vi "Tests_Window.vi"   [LabVIEW 2024]
uses:
  GLF/Window/Window.lvclass
  GLF/View/View.lvclass
  GLF/Engine/Engine.lvclass
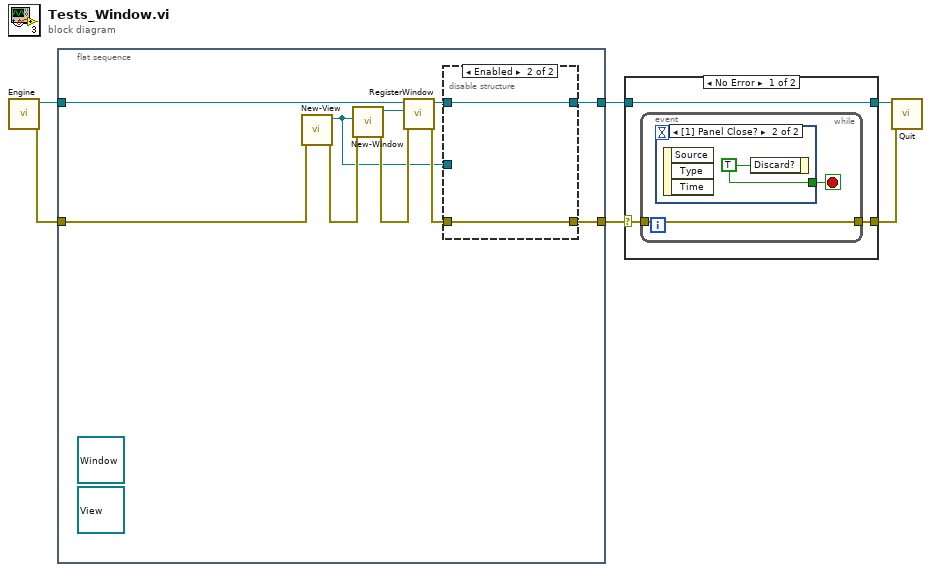
[diagram p0: block diagram]
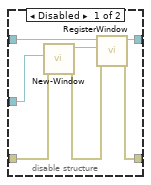
[diagram p2: hidden frame]
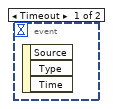
[diagram p3: hidden frame]
diagram:
  n1 = call "Engine.vi"() -> ("error out"=w5:errorcluster, "Engine"=w1:refnum<class "Engine.lvclass">)  [unwired: 10 in]
  n2 = flat-sequence {
    tunnel: w5 -> [w16]
    tunnel: [w8] -> w4
    tunnel: [w10] -> w2
    tunnel: w1 -> [w12]
    frame #0 {
      (unwired) refnum<class "View.lvclass"> refnum ("GLF.lvlib:View.lvclass")
      (unwired) refnum<class "Window.lvclass"> refnum ("GLF.lvlib:Window.lvclass")
      n3 = call "New-View.vi"("error in (no error)"=w16) -> ("error out"=w15:errorcluster, "View out"=w7:refnum<class "View.lvclass">)  [unwired: 9 in]
      n4 = call "New-Window.vi"("error in (no error)"=w15, "View"=w7) -> ("error out"=w14:errorcluster, "Window"=w13:refnum<class "Window.lvclass">)  [unwired: 8 in]
      n5 = call "RegisterWindow.vi"("error in (no error)"=w14, "Window"=w13, "Engine in"=w12) -> ("error out"=w9:errorcluster, "Engine out"=w11:refnum<class "Engine.lvclass">)  [unwired: 7 in]
      n6 = disable-structure shown="Enabled" {
        disable-tunnel: w11 -> [w23 w25]
        disable-tunnel: [w22 w25] -> w10
        disable-tunnel: w9 -> [w20 w24]
        disable-tunnel: [w18 w24] -> w8
        disable-tunnel: w7 -> [w17 _]
        frame Disabled {
          n7 = call "New-Window.vi"("error in (no error)"=w20, "View"=w17) -> ("error out"=w19:errorcluster, "Window"=w21:refnum<class "Window.lvclass">)  [unwired: 8 in]
          n8 = call "RegisterWindow.vi"("error in (no error)"=w19, "Window"=w21, "Engine in"=w23) -> ("error out"=w18:errorcluster, "Engine out"=w22:refnum<class "Engine.lvclass">)  [unwired: 7 in]
        }
        frame Enabled {
        }
      }
    }
  }
  n9 = case shown="No Error" w4 {
    selector: w4 -> [w27 w32]
    tunnel: [w28 w32] -> w6
    tunnel: [w26 w33] -> w3
    tunnel: w2 -> [w26 w33]
    frame No Error {
      n10 = while {
        tunnel: w27 -> [w29]
        tunnel: [w29] -> w28
        stop <- w30 stop-if-true
        n11 = event shown="[1] Panel Close?" {
          selector: _ -> [_ _]
          dyn-events: _ -> [_ _]
          timeout: _ -> [_ _]
          tunnel: [_ w31] -> w30
          event Timeout {
            n12 = event-data() -> ()  [unwired: 1 in, 3 out]
          }
          event Panel Close? {
            w31 = TRUE ("Discard?")
            n13 = event-data() -> ()  [unwired: 1 in, 3 out]
            n14 = event-data("Discard?"=w31) -> ()  [unwired: 1 in, 1 out]
          }
        }
      }
    }
    frame Error {
    }
  }
  n15 = call "Quit.vi"("error in (no error)"=w6, "Engine in"=w3) -> ()  [unwired: 9 in, 1 out]
